vi "KundtsTube.vi"() -> ()   [LabVIEW 2014]
panel:
  in  "Array Parameters":T1 {"Spacing" items=["Linear", "Logarithmic"]}
  in  "Tab Control":enum32{"Sweep", "Single"}(tab)
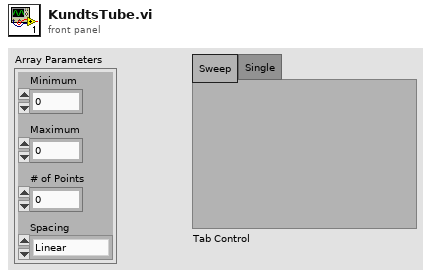
[diagram p1: front panel]
types:
  T1 = cluster{"Minimum":dbl, "Maximum":dbl, "# of Points":dbl, "Spacing":u16}
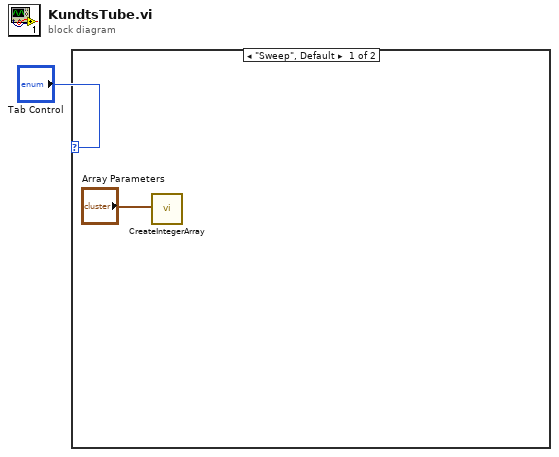
[diagram p0: block diagram]
diagram:
  n1 = case shown="\"Sweep\", Default" "Tab Control" {
    frame "Sweep", Default {
      n2 = call "CreateIntegerArray.vi"("Array Parameters"="Array Parameters") -> ()  [unwired: 10 in, 1 out]
    }
    frame "Single" {
    }
  }
